vi "editDialog.vi"(0 "reference":refnum<class "SegmentedLineEdge.lvclass">, 5 "error in (no error)":errorcluster) -> (14 "reference out":refnum<class "SegmentedLineEdge.lvclass">, 15 "cancel":bool, 19 "error out":errorcluster)   [LabVIEW 2016, in "SegmentedLineEdge.lvclass"]
doc: "Edit Dialog"
uses:
  <resource>/Framework/Providers/Open_GDS/UML/SegmentedLineEdge_class/SegmentedLineEdge.lvclass
  <resource>/Framework/Providers/Open_GDS/UML/ContextHelp/ContextHelp_HelpTexts.ctl
panel:
  in  "Help":bool
  in  "options":cluster{"include":bool, "extend":bool}
  in  "Label":string
  in  "Cancel Button":bool
  in  "OK Button":bool
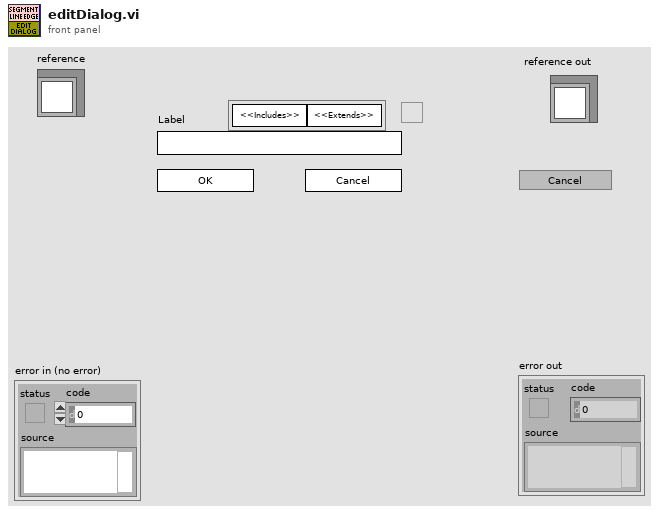
[diagram p1: front panel]
types:
  T1 = typedef "ContextHelp_HelpTexts.ctl" = enum16{"None(Hide)", "Default", "Help", "Welcome", "GettingStarted", "ClassDiagram_Help", "SequenceDiagram_Help", "UseCaseDiagram_Help", "BSelect", "BClass", "BInterface", "BPackage", "BNote", "BDependency", "BInheritance", "BInterfaceImplementation", "BAssociation", "BAggregation", "BCompAggregation", "BNoteConnector", "BObject", "BActionBar", "BCall", "BSystem", "BActor", "BUseCase", "BGeneralization", "BIncludes", "BExtends", "BUseCaseDiagramAssociation", "ClassRelationshipEdge editDialog_Bent Style", "ClassRelationshipEdge editDialog_RelationType", "ClassRelationshipEdge editDialog_Reverse association", "ClassRelationshipEdge editDialog_Start label", "ClassRelationshipEdge editDialog_Middle label", "ClassRelationshipEdge editDialog_End label", "UMLEditor reversedEngineering_Pathes", "ReversedEngineering StateReverseDialog_Help", "ReversedEngineering StateQueuedSettings_Help", "UMLEditor reversedEngineering_AddTopVIs", "UMLEditor reversedEngineering_AddClasses", "UMLEditor reversedEngineering_AddDirs", "UMLEditor reversedEngineering_Recursively", "UMLEditor reversedEngineering_Remove", "UMLEditor reversedEngineering_ClearList", "UMLEditor reversedEngineering_HideSubAss", "UMLEditor reversedEngineering_CreateTypes", "UMLEditor reversedEngineering_OnlyInheritance", "UMLEditor reversedEngineering_CreateApplication", "UMLEditor reversedEngineering_OK", "UMLEditor reversedEngineering_Cancel", "UMLEditor reversedEngineering_Help", "UMLEditor createWizardScriptFile_ScriptfilePath", "UMLEditor createWizardScriptFile_ClassPath", "UMLEditor createWizardScriptFile_Use", "UMLEditor createWizardScriptFile_PrivateDirName", "UMLEditor createWizardScriptFile_DirAppend", "UMLEditor createWizardScriptFile_Separator Character", "UMLEditor createWizardScriptFile_OK", "UMLEditor createWizardScriptFile_Cancel", "UMLEditor createWizardScriptFile_Help", "ClassNode editDialog_Class Name", "InterfaceNode editDialog_Class Name", "ClassNode editDialog_Attribute", "ClassNode editDialog_Methods", "InterfaceNode editDialog_Methods", "ClassNode editDialog_connection", "InterfaceNode editDialog_connection", "ClassNode editDialog_StereoType", "ClassNode editDialog_ShowAttrib", "ClassNode editDialog_ShowMethods", "ClassNode editDialog_ClassPath", "ClassNode editDialog_AddAttribute", "ClassNode editDialog_AddMethod", "InterfaceNode editDialog_AddMethod", "ClassNode AttributeGuide_AttributeName", "ClassNode AttributeGuide_Array?", "ClassNode AttributeGuide_Data Type", "ClassNode AttributeGuide_RefName", "ClassNode AttributeGuide_Preview", "ClassNode AttributeGuide_OK", "ClassNode AttributeGuide_Cancel", "ClassNode MethodGuide_Visibility", "ClassNode MethodGuide_Method Name", "ClassNode MethodGuide_Preview", "ClassNode MethodGuide_OK", "ClassNode MethodGuide_Cancel", "CallNode EditCallProperties_AllButtons", "ObjectNode EditObjectlProperties_AllButtons", "ActorNode EditActorProperties_AllButtons", "UseCaseRelationshipNode EditUseCaselProperties_AllButtons", "UseCaseNode EditUseCaselProperties_AllButtons", "SystemNode EditSystemProperties_AllButtons", "ReversedEngineering UpdateAttributes_AllButtons", "StateNode editDialog_AllButtons", "StateTransition editDialog_AllButtons", "ArrangeNodes Main_Picture", "ArrangeNodes Main_Zoom", "ArrangeNodes Main_Auto Zoom", "ArrangeNodes Main_shorten", "ArrangeNodes Main_Min Length", "ArrangeNodes Main_Max Length", "ArrangeNodes Main_increase", "ArrangeNodes Main_decrease", "ArrangeNodes Main_Shake", "ArrangeNodes Main", "BState", "BInitialState", "BFinalState", "BStateTransition", "StateDiagram_Help", "StateDiagram_PropertiesAllButtons", "ReversedEngineering StateReverseDialog_ClearStates", "ReversedEngineering StateReverseDialog_UseQueuedStateMachines", "ReversedEngineering StateReverseDialog_QueuedSettings", "ReversedEngineering StateReverseDialog_SearchForVIs", "ReversedEngineering StateReverseDialog_SearchCriteria", "OptionsDialog_ClassBasePath", "OptionsDialog_VIPath", "OptionsDialog_ApplicationPath", "OptionsDialog_WizDir", "OptionsDialog_IniFilePath", "OptionsDialog_DefineColors", "OptionsDialog_Help", "OptionsDialog_CreateTypes", "ClassRelationshipEdge editDialog_SplitWire"}
  T2 = typedef "SegmentedLineEdge.lvclass/ObjectAttributes.ctl" = cluster{"lineStyle":refnum<class "LineStyle.lvclass">, "startArrowHead":refnum<class "ArrowHead.lvclass">, "endArrowHead":refnum<class "ArrowHead.lvclass">, "startLabel":string, "midLabel":string, "endLabel":string, "MidLabelOffset":T3, "SplitWire":bool}
  T3 = typedef "Point Point2D.ctl" = cluster{"x":dbl, "y":dbl}
  T4 = typedef "ContextHelp_ShowType.ctl" = cluster{"Header":string, "Picture":picture, "Text":string}
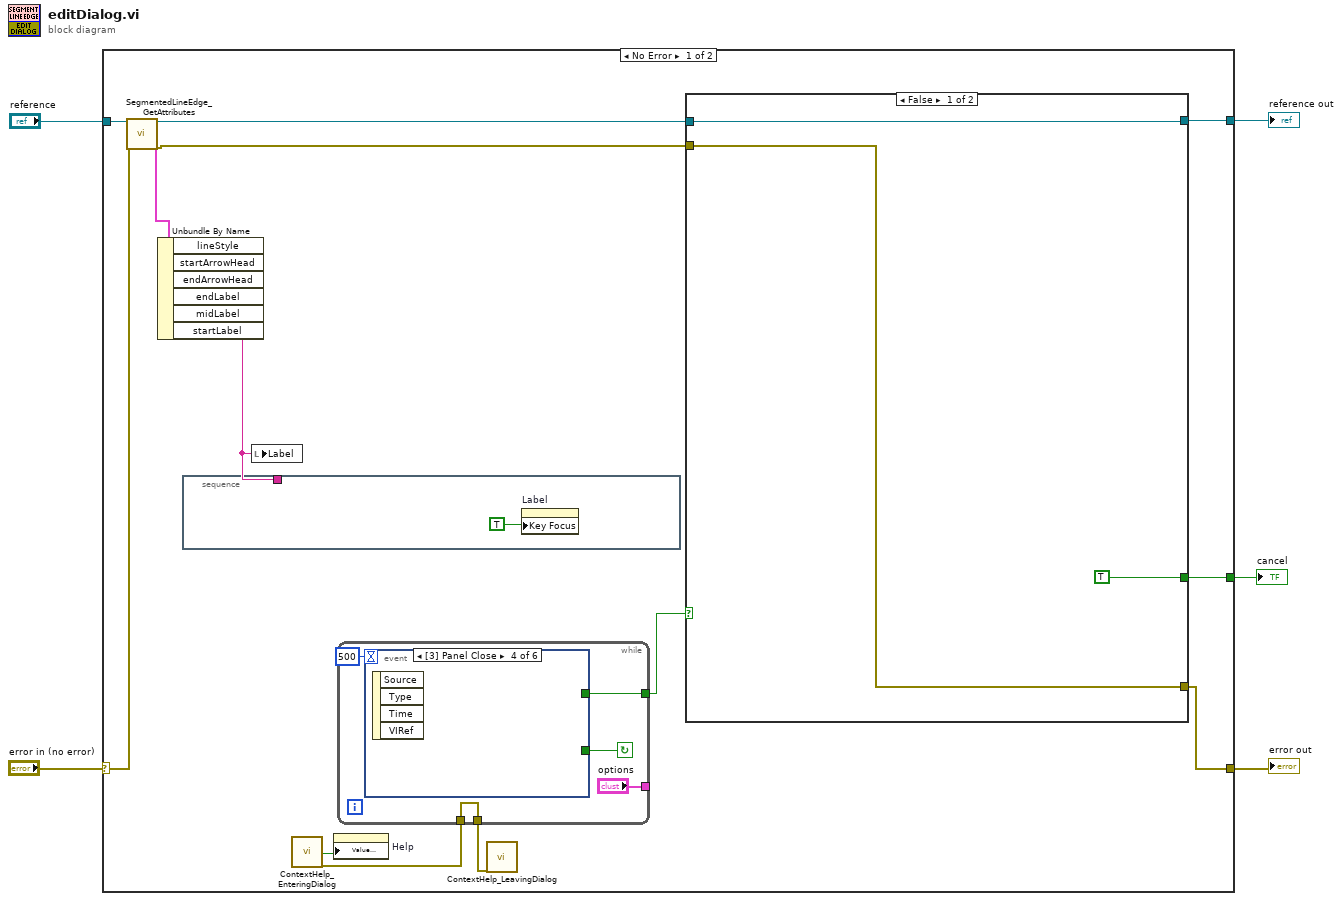
[diagram p0: block diagram]
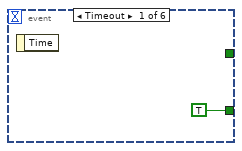
[diagram p2: hidden frame]
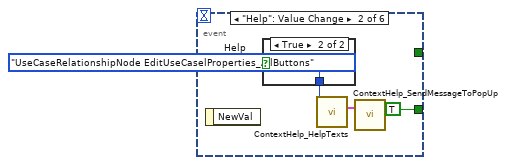
[diagram p3: hidden frame]
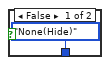
[diagram p4: hidden frame]
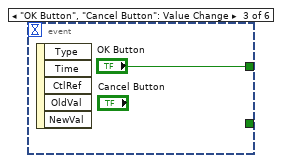
[diagram p5: hidden frame]
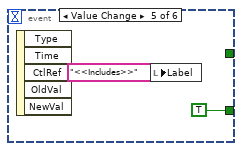
[diagram p6: hidden frame]
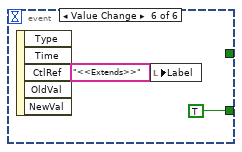
[diagram p7: hidden frame]
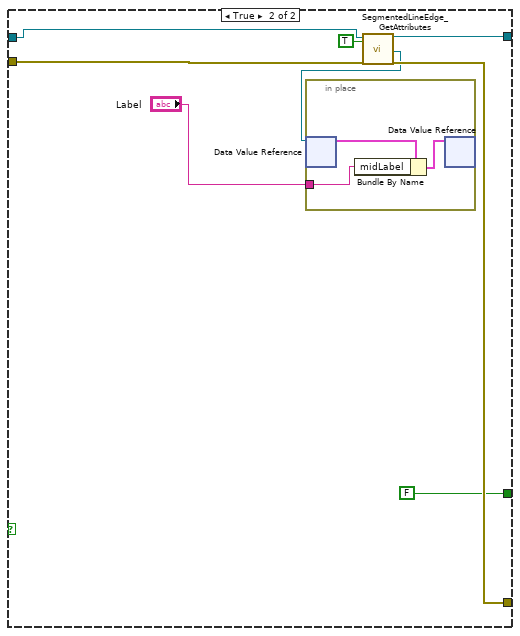
[diagram p8: hidden frame]
diagram:
  n1 = case shown="No Error" "error in (no error)" {
    selector: "error in (no error)" -> [w14 w51]
    tunnel: "reference" -> [w15 w52]
    tunnel: [w18 w51] -> w3
    tunnel: [w17 w52] -> w2
    tunnel: [w11 _] -> w1
    frame No Error {
      n2 = call <resource>:"SegmentedLineEdge_GetAttributes.vi"("reference in"=w15, "error in (no error)"=w14) -> ("reference out"=w16:refnum<class "SegmentedLineEdge.lvclass">, "Data"=w6:T2, "error out"=w10:errorcluster)  [unwired: 1 in, 14 out]
      n3 = Unbundle By Name(w6) -> ("midLabel"=w12:string)  [unwired: 5 out]
      n4 = stacked-sequence {
        tunnel: w12 -> [_]
        frame #0 {
          n5 = property on="Label" class="Str"("Key Focus"=TRUE) -> ()  [unwired: 2 in, 2 out]
        }
      }
      n6 = local write "Label"(w12) -> ()
      n7 = call <resource>:"ContextHelp_EnteringDialog.vi"() -> ("HelpStatus"=w9:bool, "error out"=w7:errorcluster)  [unwired: 3 in, 15 out]
      n8 = property on="Help" class="Bool (strict)"("Value (Signaling)"=w9) -> ()  [unwired: 2 in, 2 out]
      n9 = while {
        tunnel: [w23] -> w13
        tunnel: ["options"] -> _
        tunnel: [w19] -> w8
        tunnel: w7 -> [w19]
        stop <- w22 continue-if-true
        n10 = event shown="[3] Panel Close" {
          selector: _ -> [_ _ _ _ _ _]
          dyn-events: _ -> [_ _ _ _ _ _]
          timeout: 500 -> [_ _ _ _ _ _]
          tunnel: [_ _ "OK Button" _ _ _] -> w23
          tunnel: [TRUE TRUE _ _ TRUE TRUE] -> w22
          event Timeout {
            n11 = event-data() -> ()  [unwired: 2 out]
          }
          event "Help": Value Change {
            n12 = event-data() -> ()  [unwired: 2 out]
            n13 = case shown="True" "Help" {
              tunnel: [ContextHelp_HelpTexts."None(Hide)" ("HelpText") ContextHelp_HelpTexts."UseCaseRelationshipNode EditUseCaselProperties_AllButtons" ("HelpText")] -> w27
              frame False {
              }
              frame True {
              }
            }
            n14 = call <resource>:"ContextHelp_HelpTexts.vi"("HelpText (enum or string)"=w27) -> ("HelpOut"=w28:T4)  [unwired: 18 out]
            n15 = call <resource>:"ContextHelp_SendMessageToPopUp.vi"("PopUpMessage"=w28) -> ()  [unwired: 2 in, 17 out]
          }
          event "OK Button", "Cancel Button": Value Change {
            n16 = event-data() -> ()  [unwired: 6 out]
          }
          event Panel Close {
            n17 = event-data() -> ()  [unwired: 5 out]
          }
          event "options.include": Value Change {
            n18 = event-data() -> ()  [unwired: 6 out]
            n19 = local write "Label"("<<Includes>>" ("Label")) -> ()
          }
          event "options.extend": Value Change {
            n20 = event-data() -> ()  [unwired: 6 out]
            n21 = local write "Label"("<<Extends>>" ("Label")) -> ()
          }
        }
      }
      n22 = call <resource>:"ContextHelp_LeavingDialog.vi"("error in (no error)"=w8) -> ()  [unwired: 2 in, 17 out]
      n23 = case shown="False" w13 {
        tunnel: [w36 w46] -> w18
        tunnel: [w38 w45] -> w17
        tunnel: w16 -> [w38 w44]
        tunnel: [TRUE ("Key Focus") FALSE ("Key Focus")] -> w11
        tunnel: w10 -> [w36 w42]
        frame False {
        }
        frame True {
          n24 = call <resource>:"SegmentedLineEdge_GetAttributes.vi"("reference in"=w44, "OnlyGetDvrReference(False)"=TRUE, "error in (no error)"=w42) -> ("reference out"=w45:refnum<class "SegmentedLineEdge.lvclass">, "DataRef"=w40:refnum<data-value>, "error out"=w46:errorcluster)  [unwired: 13 in, 1 out]
          n25 = in-place {
            in-place-border: "Label" -> [w48]
            n26 = in-place-dvr #1(w40) -> (w49:T2)  [unwired: 1 out]
            n27 = Bundle By Name(cluster=w49, "midLabel"=w48) -> (w47:T2)
            n28 = in-place-dvr #1(w47) -> ()  [unwired: 2 out]
          }
        }
      }
    }
    frame Error {
    }
  }
  "reference out" <- w2
  "error out" <- w3
  "cancel" <- w1
